vi "SPCM_initialize.vi"() -> ()   [LabVIEW 2012]
uses:
  spcm_functions_lv10.llb/error.ctl
  spcm_functions_lv10.llb/SPC_mod_info.ctl
  spcm_functions_lv10.llb/Global_SPCM_vars.vi
  SPCM_DLL_path.vi
panel:
  out "DLL not loaded":string=" DLL not loaded  - set default DLL path in  SPCM_DLL_path.vi"
  out "DLL_path":path
  in  "New DLL mode":i16(ring) items=["Hardware mode", "Simulation of SPC130", "Simulation of SPC600", "Simulation of SPC-630", "Simulation of SPC-700", "Simulation of SPC-730", "Simulation of SPC-830", "Simulation of SPC-140", "Simulation of SPC-930", "Simulation of SPC-150", "Simulation of DPC-230", "Simulation of SPC-130-EM"]
  out "SPC module info":T1={"module type"=-1, "bus number"=-1, "slot number"=-1, "in use"=0, "init status"=-1, "base I/O addr"=0} {"bus number" min=0 max=255 step=1; "base I/O addr" format="%.0x"; "init status" min=-10 max=0 step=1; "in use" min=-1 max=1 step=1; "slot number" min=0 max=255 step=1; "module type" min=-32767 step=1}
  out "Base I/O addr":u16 format="%.0x"
  out "Slot":i16 min=0 max=255 step=1
  out "Bus":i16 min=0 max=255 step=1
  in  "Old active module":u16(ring) items=["Module 0", "Module 1", "Module 2", "Module 3", "Module 4", "Module 5", "Module 6", "Module 7"]
  in  "Old Mod No":u16(ring) items=["Module 0", "Module 1", "Module 2", "Module 3", "Module 4", "Module 5", "Module 6", "Module 7"]
  out "use_array":bool[](array[boolean])
  out "First":bool
  out "Modules in use":T2
  in  "Choose modules to use":T2={"M0"=TRUE, "M1"=TRUE, "M2"=TRUE, "M3"=TRUE, "M4"=TRUE, "M5"=TRUE, "M6"=TRUE, "M7"=TRUE}
  in  "Information":u16(ring) items=["Module 0", "Module 1", "Module 2", "Module 3", "Module 4", "Module 5", "Module 6", "Module 7"]
  in  "Choose active module":u16(ring) items=["Module 0", "Module 1", "Module 2", "Module 3", "Module 4", "Module 5", "Module 6", "Module 7"]
  out "Number of used modules":i16 min=0 max=4
  in  "Force use":i16 min=0 max=1
  out "Choose modules":T3={"M0"=1, "M1"=1, "M2"=1, "M3"=1, "M4"=1, "M5"=1, "M6"=1, "M7"=1} {"M7" min=0 max=1; "M6" min=0 max=1; "M5" min=0 max=1; "M4" min=0 max=1; "M3" min=0 max=1; "M2" min=0 max=1; "M1" min=0 max=1; "M0" min=0 max=1}
  out "Current mode value":i16
  in  "change mode":bool
  in  "stop":bool
  out "Type":string
  out "Ini message":string
  out "Current DLL mode":string
  out "SPC error":T4
  out "prompt":string
  out "Default name":string="spc400.ini"
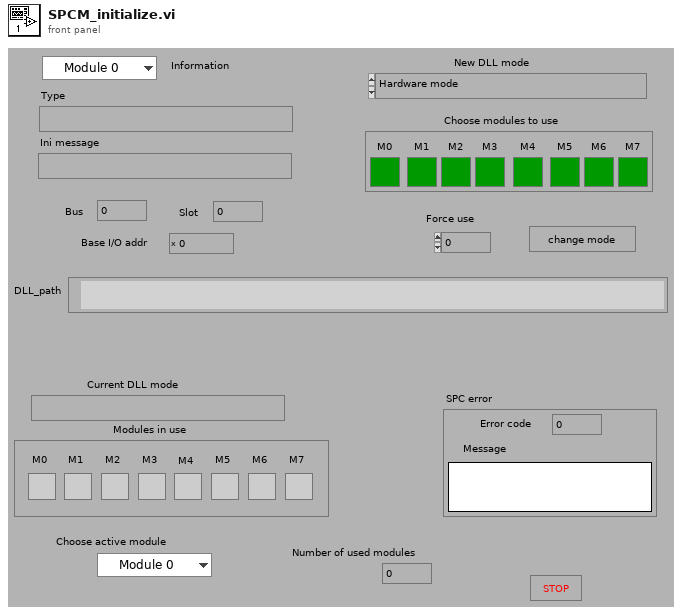
[diagram p1: front panel]
types:
  T1 = typedef "SPC_mod_info.ctl" = cluster{"module type":i16, "bus number":i16, "slot number":i16, "in use":i16, "init status":i16, "base I/O addr":u16}
  T2 = cluster{"M0":bool, "M1":bool, "M2":bool, "M3":bool, "M4":bool, "M5":bool, "M6":bool, "M7":bool}
  T3 = cluster{"M0":i32, "M1":i32, "M2":i32, "M3":i32, "M4":i32, "M5":i32, "M6":i32, "M7":i32}
  T4 = typedef "error.ctl" = cluster{"Error code":i16, "Message":string}
  T5 = cluster{"Base Address":u16, "Init status":i16, "CFD Limit Low [mV]":sgl, "CFD Limit High [mV]":sgl, "CFD ZC Level [mV]":sgl, "CFD Holdoff [ns]":sgl, "SYNC ZC Level [mV]":sgl, "SYNC Holdoff [ns]":sgl, "SYNC Threshold [mV]":sgl, "TAC Range [ns]":sgl, "SYNC Freq Divider":i16, "TAC Gain":i16, "TAC Offset [%]":sgl, "TAC Limit Low [%]":sgl, "TAC Limit High [%]":sgl, "ADC Resolution":i16, "Ext Latch Delay":i16, "Collection Time [s]":sgl, "Display Time [s]":sgl, "Repeat Time [s]":sgl, "Stop on Time":i16, "Stop on Overflow":i16, "Dither Range":i16, "Count Increment":i16, "Memory Bank":i16, "Dead Time Compensation":i16, "Scan Control":u16, "Routing Mode":i16, "TAC Enable Hold":sgl, "Slot No of PCI Module":i16, "Operation Mode":u16, "Scan Size X":u32, "Scan Size Y":u32, "Scan Routing Size X ":u32, "Scan Routing Size Y":u32, "Scan Flyback":u32, "Scan Borders":u32, "Scan Polarity":u16, "Pixel Clock Source":u16, "Line Compression":u16, "External Trigger Condition":u16, "Pixel Time [s]":sgl, "External pixel clock divider":u32, "Rate Counting Time":sgl, "Macro Time Clock  ":i16, "ADD Signal Source":i16, "Test EEPROM":i16, "ADC Zoom":i16, "Image Size X":u32, "Image Size Y":u32, "Image Routing Size X":u32, "Image Routing Size Y":u32, "XY Gain":i16, "Master Clock":i16, "ADC Sample Delay":i16, "Detector Type":i16, "X Axis Type":i16, "Channel enable ( DPC-230)":u32, "Channel slope ( DPC-230)":u32, "Channel spec_no ( DPC-230)":u32}
  T6 = typedef "mem_config.ctl" = cluster{"max_block_no":i32, "blocks_per_frame":i32, "frames_per_page":i32, "maxpage":i32, "block_length":i16}
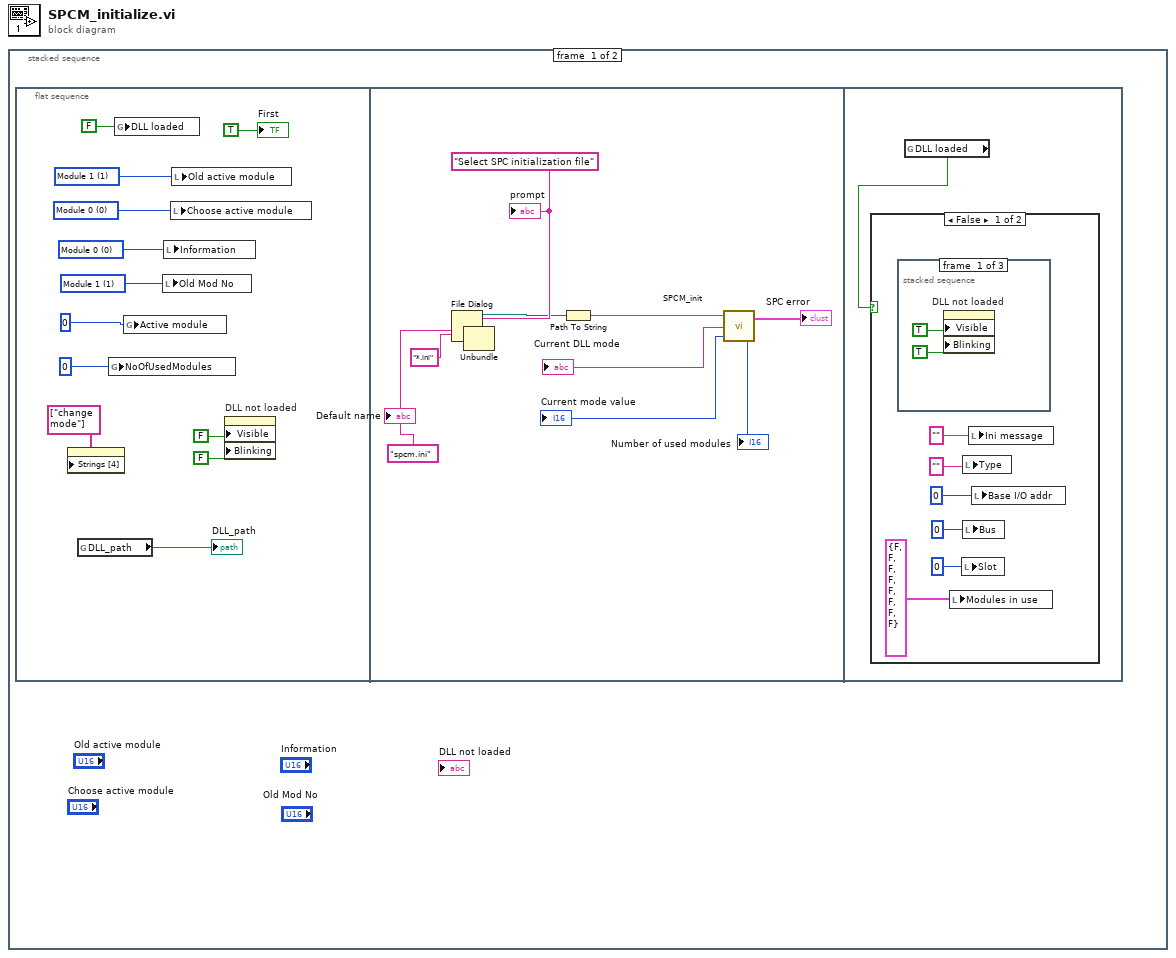
[diagram p0: block diagram]
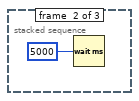
[diagram p2: hidden frame]
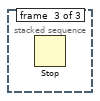
[diagram p3: hidden frame]
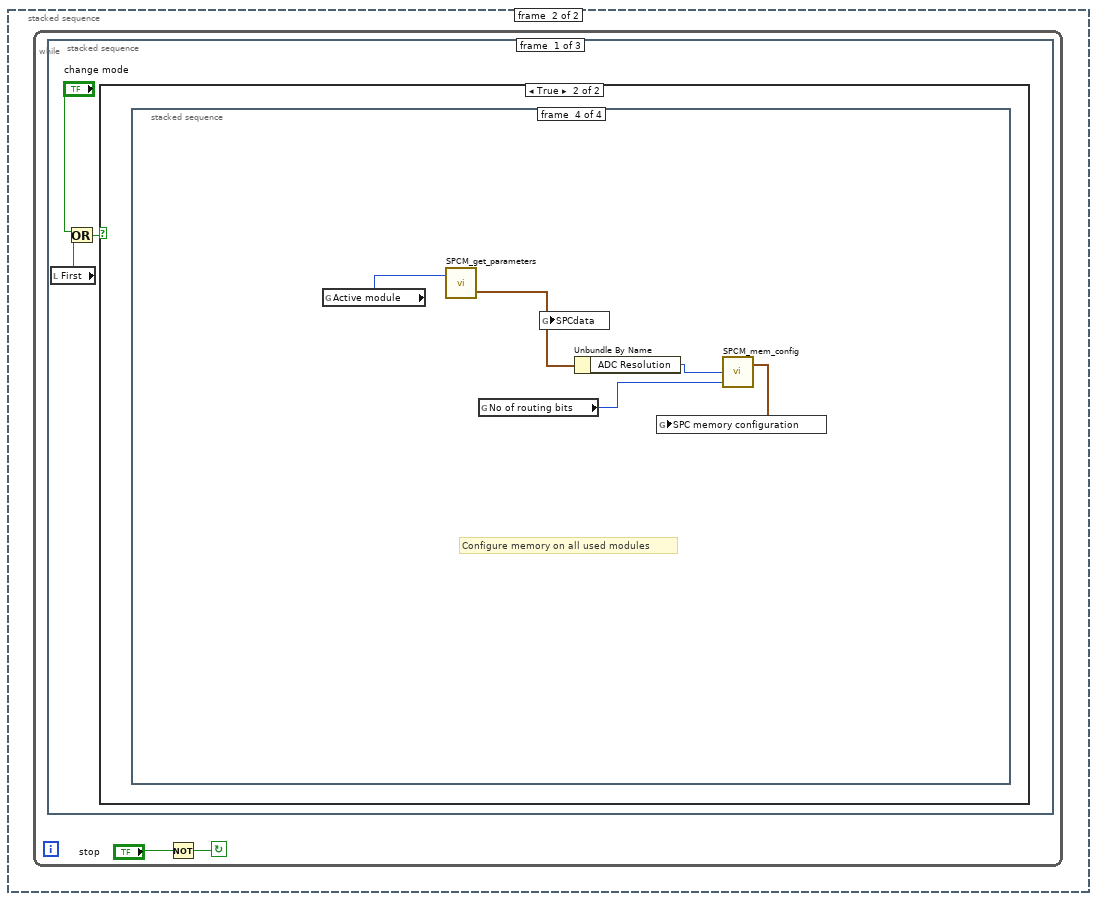
[diagram p5: hidden frame]
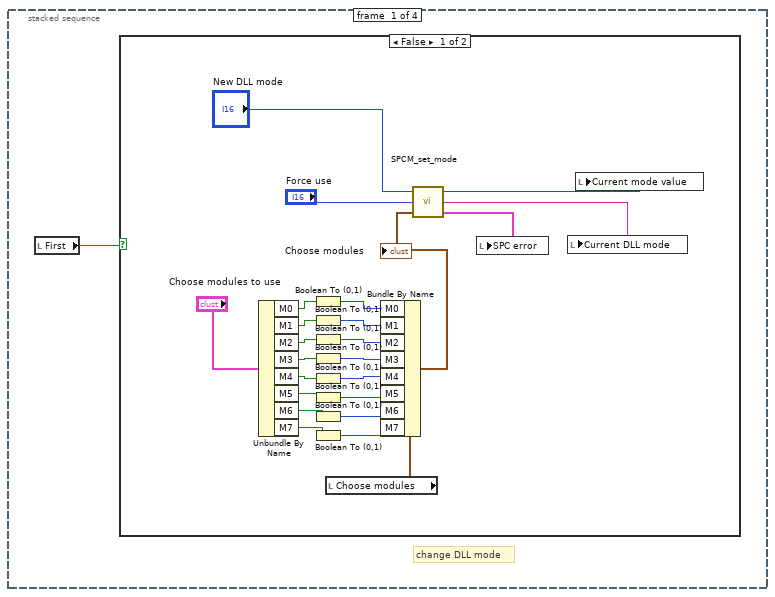
[diagram p7: hidden frame]
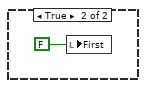
[diagram p8: hidden frame]
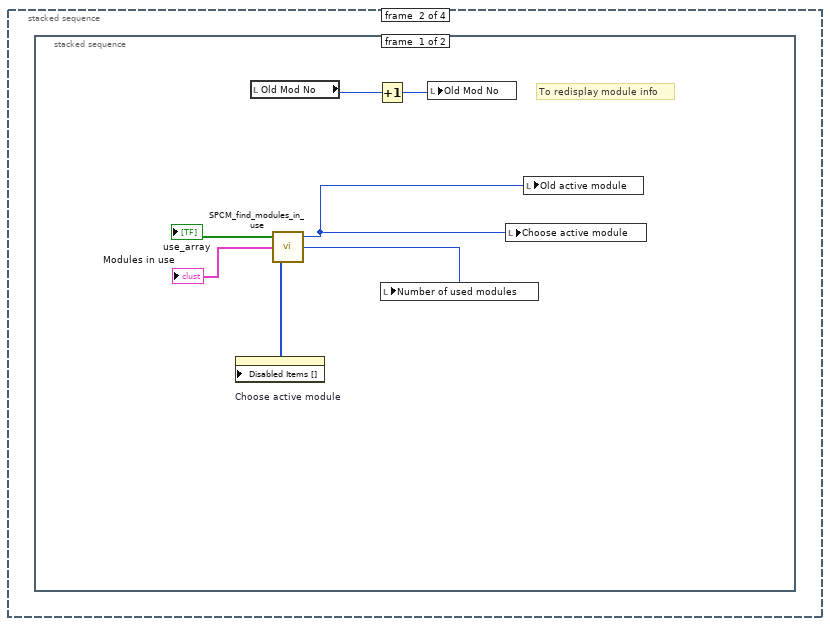
[diagram p9: hidden frame]
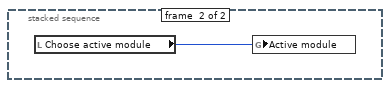
[diagram p10: hidden frame]
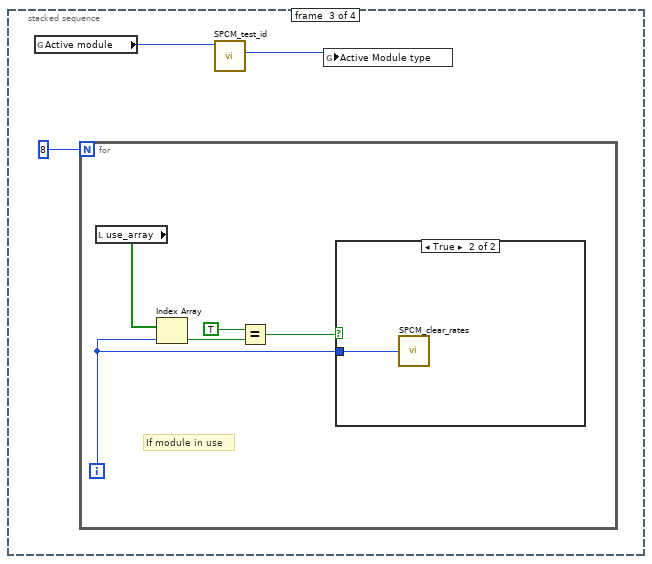
[diagram p11: hidden frame]
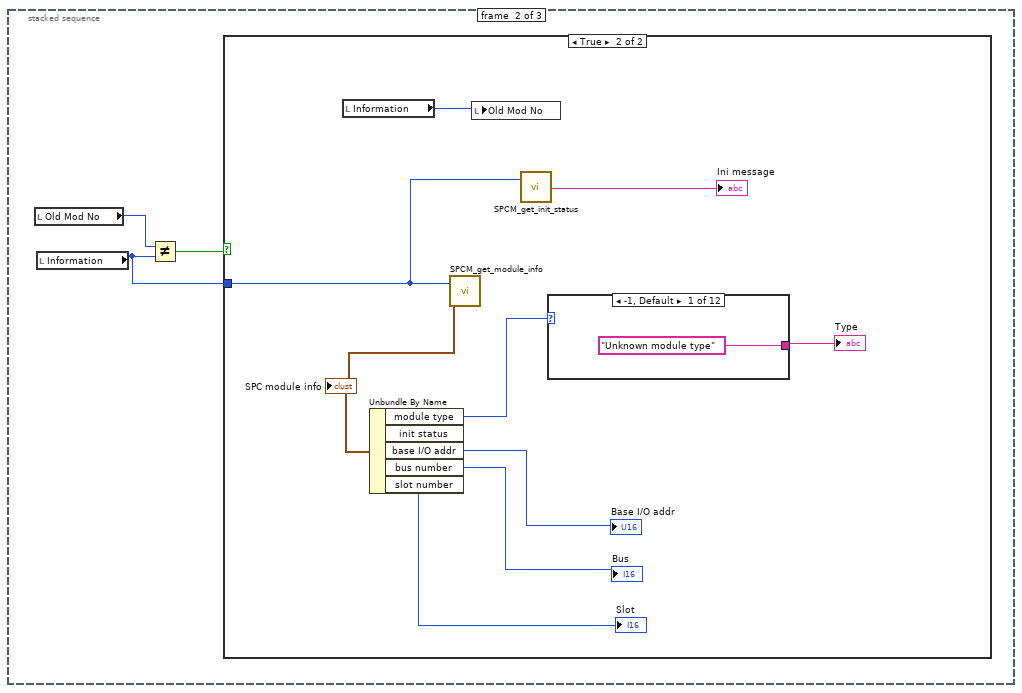
[diagram p13: hidden frame]
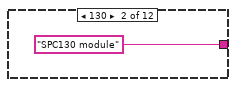
[diagram p15: hidden frame]
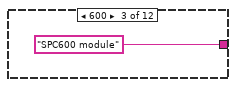
[diagram p16: hidden frame]
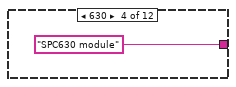
[diagram p17: hidden frame]
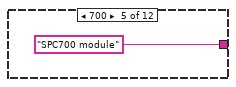
[diagram p18: hidden frame]
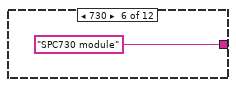
[diagram p19: hidden frame]
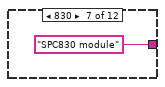
[diagram p20: hidden frame]
diagram:
  n1 = stacked-sequence {
    frame #0 {
      n2 = flat-sequence {
        frame #0 {
          w11 = u16 1 items=["Module 0", "Module 1", "Module 2", "Module 3", "Module 4", "Module 5", "Module 6", "Module 7"] ("Old active module")
          w10 = u16 1 items=["Module 0", "Module 1", "Module 2", "Module 3", "Module 4", "Module 5", "Module 6", "Module 7"] ("Old Mod No")
          w9 = u16 0 items=["Module 0", "Module 1", "Module 2", "Module 3", "Module 4", "Module 5", "Module 6", "Module 7"] ("Choose active module")
          w8 = u16 0 items=["Module 0", "Module 1", "Module 2", "Module 3", "Module 4", "Module 5", "Module 6", "Module 7"] ("Information")
          n3 = property on="change mode" class="Bool"("Strings [4]"=string[] ["change mode"]) -> ()  [unwired: 2 in, 2 out]
          n4 = global read "SPCM_DLL_path.vi" "DLL_path"() -> (→"DLL_path":path)
          n5 = global write "Global_SPCM_vars.vi" "NoOfUsedModules"(i16 0 ("NoOfUsedModules")) -> ()
          n6 = global write "SPCM_DLL_path.vi" "DLL loaded"(FALSE ("DLL loaded")) -> ()
          n7 = global write "Global_SPCM_vars.vi" "Active module"(i16 0 ("Active module")) -> ()
          n8 = local write "Old Mod No"(w10) -> ()
          n9 = local write "Information"(w8) -> ()
          n10 = local write "Choose active module"(w9) -> ()
          n11 = local write "Old active module"(w11) -> ()
          n12 = property on="DLL not loaded" class="Str"("Visible"=FALSE, "Blinking"=FALSE) -> ()  [unwired: 2 in, 2 out]
          "First" <- TRUE ("First")
        }
        frame #1 {
          w20 = "spcm.ini" ("Default name")
          w16 = "Select SPC initialization file" ("prompt")
          n13 = File Dialog(6:"*.ini" ("pattern"), 7:w16, 9:w20) -> (0:w22:errorcluster, 3:w15:path)  [unwired: 4 in, 2 out]
          n14 = Unbundle(w22) -> ()  [unwired: 3 out]
          n15 = Path To String(path=w15) -> (string=w14:string)
          n16 = call "SPCM_init.vi"("Ini file name"=w14) -> ("Number of used modules"=→"Number of used modules":i16, "SPC error"=→"SPC error":cluster{"Error code":i16, "Message":string}, "Current mode value"=→"Current mode value":i16, "Current DLL mode"=→"Current DLL mode":string)
          "prompt" <- w16
          "Default name" <- w20
        }
        frame #2 {
          n17 = global read "SPCM_DLL_path.vi" "DLL loaded"() -> (w23:bool)
          n18 = case shown="False" w23 {
            frame False {
              n19 = stacked-sequence {
                frame #0 {
                  n20 = property on="DLL not loaded" class="Str"("Visible"=TRUE, "Blinking"=TRUE) -> ()  [unwired: 2 in, 2 out]
                }
                frame #1 {
                  n21 = Wait (ms)(milliseconds to wait=u32 5000) -> ()  [unwired: 1 out]
                }
                frame #2 {
                  n22 = Stop() -> ()  [unwired: 1 in]
                }
              }
              n23 = local write "Modules in use"(T2 {"M0"=FALSE, "M1"=FALSE, "M2"=FALSE, "M3"=FALSE, "M4"=FALSE, "M5"=FALSE, "M6"=FALSE, "M7"=FALSE} ("Modules in use")) -> ()
              n24 = local write "Slot"(i16 0 ("Slot")) -> ()
              n25 = local write "Type"("" ("Type")) -> ()
              n26 = local write "Bus"(i16 0 ("Bus")) -> ()
              n27 = local write "Ini message"("" ("Ini message")) -> ()
              n28 = local write "Base I/O addr"(u16 0 ("Base I/O addr")) -> ()
            }
            frame True {
            }
          }
        }
      }
    }
    frame #1 {
      n29 = while {
        stop <- w33 continue-if-true
        n30 = stacked-sequence {
          frame #0 {
            n31 = local read "First"() -> (w36:bool)
            n32 = Or(x="change mode", y=w36) -> (x .or. y?=w35:bool)
            n33 = case shown="True" w35 {
              frame False {
              }
              frame True {
                n34 = stacked-sequence {
                  frame #0 {
                    # "change DLL mode"
                    n35 = local read "First"() -> (w38:bool)
                    n36 = case shown="False" w38 {
                      frame False {
                        n37 = Unbundle By Name("Choose modules to use") -> ("M0"=w58:bool, "M1"=w57:bool, "M2"=w56:bool, "M3"=w55:bool, "M4"=w48:bool, "M5"=w46:bool, "M6"=w43:bool, "M7"=w42:bool)
                        n38 = Boolean To (0,1)(Boolean=w58) -> (0, 1=w54:i16)
                        n39 = Boolean To (0,1)(Boolean=w57) -> (0, 1=w53:i16)
                        n40 = Boolean To (0,1)(Boolean=w56) -> (0, 1=w52:i16)
                        n41 = Boolean To (0,1)(Boolean=w55) -> (0, 1=w51:i16)
                        n42 = Boolean To (0,1)(Boolean=w48) -> (0, 1=w47:i16)
                        n43 = Boolean To (0,1)(Boolean=w46) -> (0, 1=w45:i16)
                        n44 = Boolean To (0,1)(Boolean=w43) -> (0, 1=w44:i16)
                        n45 = Boolean To (0,1)(Boolean=w42) -> (0, 1=w41:i16)
                        n46 = local read "Choose modules"() -> (w49:T3)
                        n47 = Bundle By Name(cluster=w49, "M0"=w54, "M1"=w53, "M2"=w52, "M3"=w51, "M4"=w47, "M5"=w45, "M6"=w44, "M7"=w41) -> (w50:T3)
                        "Choose modules" <- w50
                        n48 = call "SPCM_set_mode.vi"("Modules in use"=w50, "Force use"="Force use", "New mode"="New DLL mode") -> ("SPC error"=w60:cluster{"Error code":i16, "Message":string}, "Mode text"=w61:string, "Mode value"=w40:i16)
                        n49 = local write "SPC error"(w60) -> ()
                        n50 = local write "Current DLL mode"(w61) -> ()
                        n51 = local write "Current mode value"(w40) -> ()
                      }
                      frame True {
                        n52 = local write "First"(FALSE ("First")) -> ()
                      }
                    }
                  }
                  frame #1 {
                    n53 = stacked-sequence {
                      frame #0 {
                        # "To redisplay module info"
                        n54 = local read "Old Mod No"() -> (w70:u16)
                        n55 = call "SPCM_find_modules_in_use.vi"() -> ("Number of used modules"=w65:i16, "First active module"=w64:u16, "Disabled Items"=w66:i32[], "Use LEDs"=→"Modules in use":T2, "use_array"=→"use_array":bool[])  [unwired: 1 out]
                        n56 = property on="Choose active module" class="Ring (strict)"("Disabled Items []"=w66) -> ()  [unwired: 2 in, 2 out]
                        n57 = Increment(x=w70) -> (x+1=w69:u16)
                        n58 = local write "Number of used modules"(w65) -> ()
                        n59 = local write "Old Mod No"(w69) -> ()
                        n60 = local write "Choose active module"(w64) -> ()
                        n61 = local write "Old active module"(w64) -> ()
                      }
                      frame #1 {
                        n62 = local read "Choose active module"() -> (w71:u16)
                        n63 = global write "Global_SPCM_vars.vi" "Active module"(w71) -> ()
                      }
                    }
                  }
                  frame #2 {
                    n64 = global read "Global_SPCM_vars.vi" "Active module"() -> (w73:i16)
                    n65 = for {
                      N: 8 -> [_]
                      i -> [w75]
                      # "If module in use"
                      n66 = local read "use_array"() -> (w79:bool[])
                      n67 = Index Array(array=w79, index=w75) -> (element=w78:bool)
                      n68 = Equal?(x=TRUE, y=w78) -> (x = y?=w76:bool)
                      n69 = case shown="True" w76 {
                        tunnel: w75 -> [_ w80]
                        frame False {
                        }
                        frame True {
                          n70 = call "SPCM_clear_rates.vi"("Module no"=w80) -> ()  [unwired: 1 out]
                        }
                      }
                    }
                    n71 = call "SPCM_test_id.vi"("Module no"=w73) -> ("Module type code"=w74:i16)  [unwired: 2 out]
                    n72 = global write "Global_SPCM_vars.vi" "Active Module type"(w74) -> ()
                  }
                  frame #3 {
                    # "Configure memory on all used modules"
                    n73 = global read "Global_SPCM_vars.vi" "Active module"() -> (w81:i16)
                    n74 = call "SPCM_get_parameters.vi"("Module no"=w81) -> ("SPCdata"=w85:T5)  [unwired: 1 out]
                    n75 = global read "Global_SPCM_vars.vi" "No of routing bits"() -> (w82:u16)
                    n76 = global write "Global_SPCM_vars.vi" "SPCdata"(w85) -> ()
                    n77 = Unbundle By Name(w85) -> ("ADC Resolution"=w84:i16)
                    n78 = call "SPCM_mem_config.vi"("No of routing bits"=w82, "ADC resolution"=w84) -> ("SPC memory configuration"=w83:T6)  [unwired: 1 in, 1 out]
                    n79 = global write "Global_SPCM_vars.vi" "SPC memory configuration"(w83) -> ()
                  }
                }
              }
            }
          }
          frame #1 {
            n80 = local read "Old Mod No"() -> (w88:u16)
            n81 = local read "Information"() -> (w86:u16)
            n82 = Not Equal?(x=w88, y=w86) -> (x != y?=w87:bool)
            n83 = case shown="True" w87 {
              tunnel: w86 -> [_ w90]
              frame False {
              }
              frame True {
                n84 = local read "Information"() -> (w97:u16)
                n85 = call "SPCM_get_module_info.vi"("Module no"=w90) -> ("SPC module info"=w91:T1)  [unwired: 1 out]
                "SPC module info" <- w91
                n86 = Unbundle By Name(w91) -> ("module type"=w96:i16, "base I/O addr"=→"Base I/O addr":u16, "bus number"=→"Bus":i16, "slot number"=→"Slot":i16)  [unwired: 1 out]
                n87 = local write "Old Mod No"(w97) -> ()
                n88 = call "SPCM_get_init_status.vi"("Module no"=w90) -> ("Message"=→"Ini message":string)  [unwired: 1 out]
                n89 = case shown="-1, Default" w96 {
                  tunnel: ["Unknown module type" "SPC130 module" "SPC600 module" "SPC630 module" "SPC700 module" "SPC730 module" "SPC830 module" "SPC140 module" "SPC930 module" "SPC150 module" "DPC230 module" "SPC130-EM module"] -> w95
                  frame -1, Default {
                  }
                  frame 130 {
                  }
                  frame 600 {
                  }
                  frame 630 {
                  }
                  frame 700 {
                  }
                  frame 730 {
                  }
                  frame 830 {
                  }
                  frame 140 {
                  }
                  frame 930 {
                  }
                  frame 150 {
                  }
                  frame 230 {
                  }
                  frame 131 {
                  }
                }
                "Type" <- w95
              }
            }
          }
          frame #2 {
            n90 = local read "Choose active module"() -> (w112:u16)
            n91 = local read "Old active module"() -> (w110:u16)
            n92 = Not Equal?(x=w110, y=w112) -> (x != y?=w111:bool)
            n93 = case shown="True" w111 {
              frame False {
              }
              frame True {
                n94 = local read "Choose active module"() -> (w113:u16)
                n95 = global write "Global_SPCM_vars.vi" "Active module"(w113) -> ()
                n96 = local write "Old active module"(w113) -> ()
              }
            }
          }
        }
        n97 = Not(x="stop") -> (.not. x?=w33:bool)
      }
    }
  }
